vi "ImageInArray.vi"(0 "index":i32, 1 "Array":T1[](array[typedef])) -> (2 "Image":T1)   [LabVIEW 2015]
uses:
  <vilib>/vision/Image Controls.llb/IMAQ Image.ctl
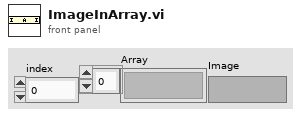
[diagram p1: front panel]
types:
  T1 = typedef "IMAQ Image.ctl" = refnum<image>
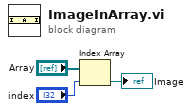
[diagram p0: block diagram]
diagram:
  n1 = Index Array(array="Array", index="index") -> (element=→"Image":T1)
